vi "ADC Knob Test State.vi"(0 "GEA2 Reference Out":refnum<k24>, 5 "Queue in":refnum<queue>, 9 "Test Results in":T1, 11 "error in (no error)":errorcluster) -> (4 ".NET Refnum out":refnum<k24>, 10 "Test Results out":T1, 15 "error out":errorcluster)   [LabVIEW 2016]
doc: "This VI performs the LED test state."
uses:
  controls/Test Results.ctl
  C:/Program Files (x86)/National Instruments/LabVIEW 2016/examples/Design Patterns/Queued Message Handler/support/QMH Fundamentals - Message Cluster.ctl
  C:/Automation/DLLs/PC Dot Net/GeaCommunication.dll
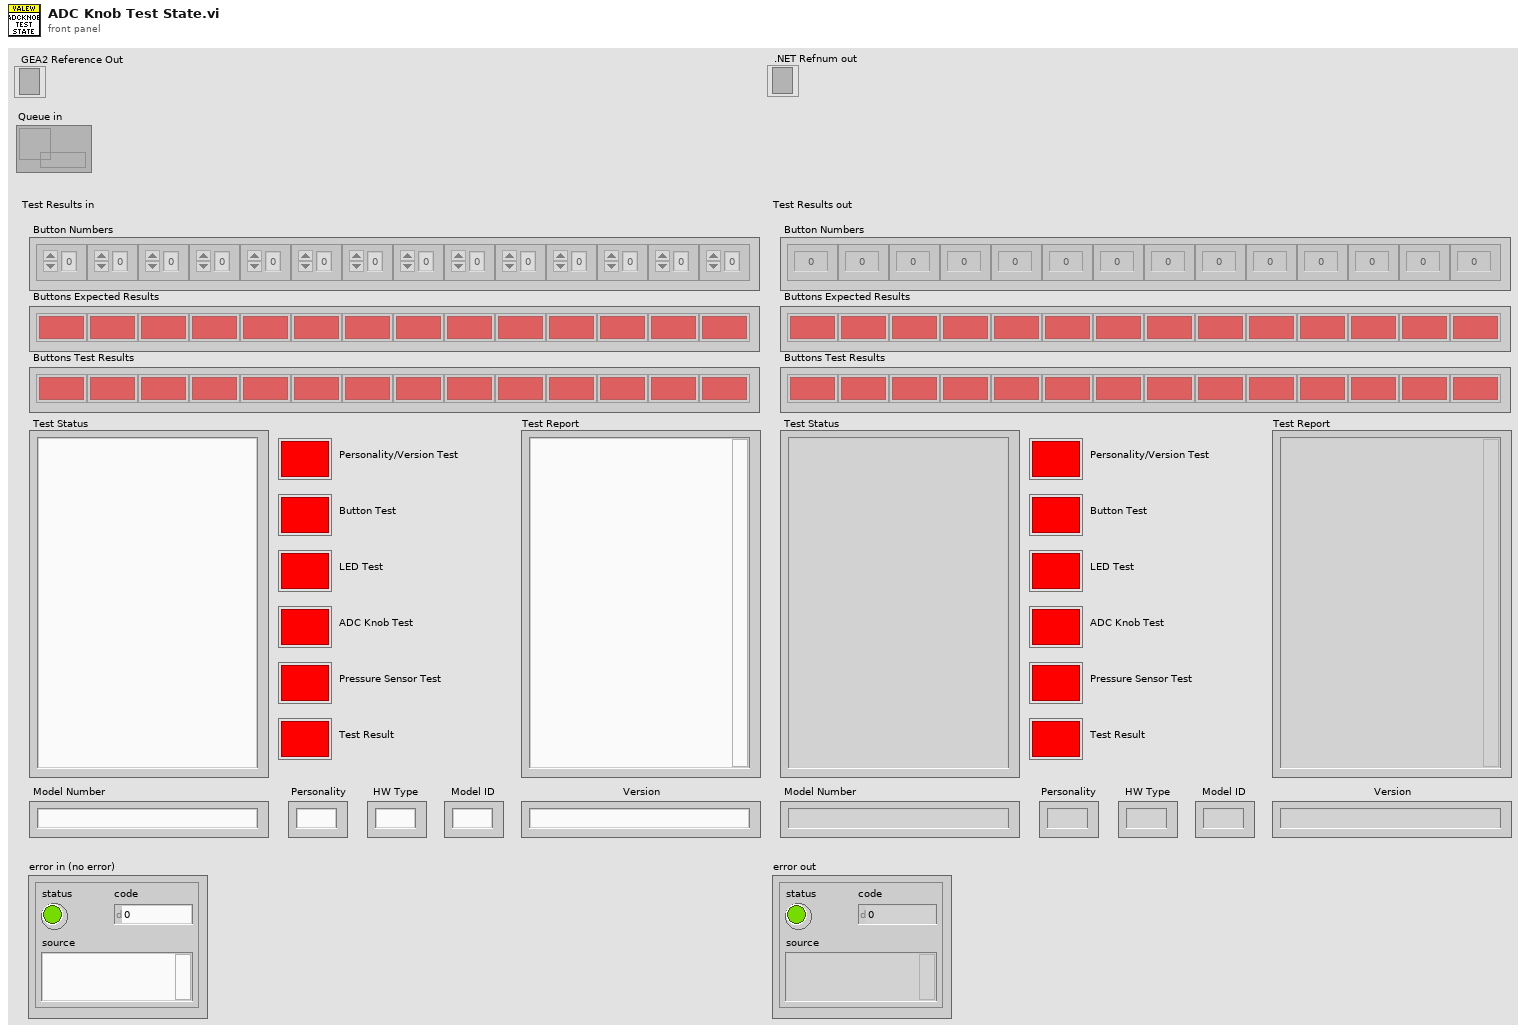
[diagram p1: front panel]
types:
  T1 = typedef "Test Results.ctl" = cluster{"Test Status":string, "Personality/Version Test ":bool, "Test Report":string, "Model Number":string, "Button Numbers":i32[], "Buttons Test Results":bool[], "Buttons Expected Results":bool[], "Model ID":string, "Personality":string, "HW Type":string, "Version":string, "Button Test":bool, "LED Test":bool, "ADC Knob Test":bool, "Pressure Sensor Test":bool, "Test Result":bool}
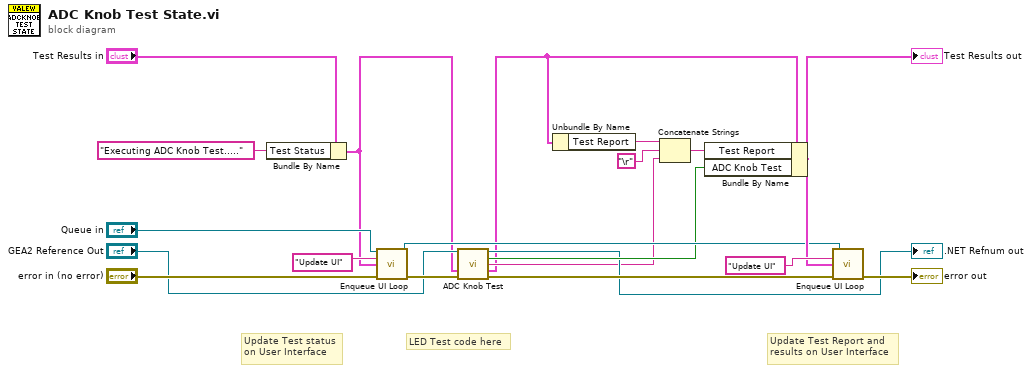
[diagram p0: block diagram]
diagram:
  # "Update Test Report and \nresults on User Interface"
  # "LED Test code here"
  # "Update Test status\non User Interface"
  n1 = Bundle By Name(cluster="Test Results in", "Test Status"="Executing ADC Knob Test.....") -> (w2:T1)
  n2 = call "Enqueue UI Loop.vi"("UI Que In"="Queue in", "Message"="Update UI", "Test Results"=w2, "error in (no error)"="error in (no error)") -> ("UI Queue Out"=w18:refnum<queue>, "error out"=w13:errorcluster)  [unwired: 10 in]
  n3 = call "ADC Knob Test.vi"("GEA2 Reference In"="GEA2 Reference Out", "Test Results in"=w2, "Error In"=w13) -> ("GEA2 Reference Out"=→".NET Refnum out":refnum<k24>, "Pass/Fail?"=w11:bool, "Report Text"=w6:string, "Test Results out"=w1:T1, "Error Out"=w16:errorcluster)  [unwired: 8 in]
  n4 = Unbundle By Name(w1) -> ("Test Report"=w3:string)
  n5 = Concatenate Strings(w3, "\r", w6) -> (w5:string)
  n6 = Bundle By Name(cluster=w1, "Test Report"=w5, "ADC Knob Test"=w11) -> (w19:T1)
  "Test Results out" <- w19
  n7 = call "Enqueue UI Loop.vi"("UI Que In"=w18, "Message"="Update UI", "Test Results"=w19, "error in (no error)"=w16) -> ("error out"=→"error out":errorcluster)  [unwired: 10 in, 1 out]
